vi "Actor Stopped.vi"(8 "error in (no error)":errorcluster, 10 "Actor's Self Q":refnum<class "Message Enqueuer.lvclass">, 11 "Monitor Data in":refnum<class "Monitor Data.lvclass">) -> (0 "error out":errorcluster, 2 "Empty?":bool, 3 "Monitor Data out":refnum<class "Monitor Data.lvclass">)   [LabVIEW 2020, in "Monitor Data.lvclass"]
doc: "Removes the actor from the data store\n\nCopyright: MGI 2016\nAuthor: Derek Trepanier"
uses:
  <vilib>/MGI/Monitored Actor/Monitor Data/Monitor Data.lvclass
  <vilib>/ActorFramework/Message Enqueuer/Message Enqueuer.lvclass
  <vilib>/MGI/Monitored Actor/Monitor Data/Monitor Data.lvclass/Monitor Data.ctl
  <vilib>/MGI/Monitored Actor/Monitor Data/Actor Data.ctl
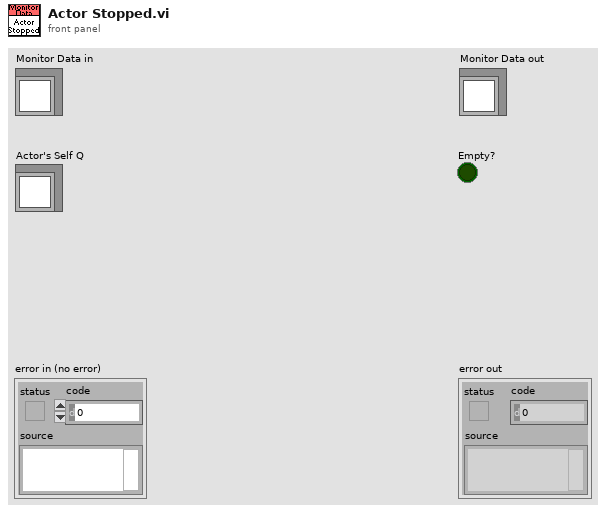
[diagram p1: front panel]
types:
  T1 = typedef "Monitor Data.lvclass/Actor Data.ctl" = cluster{"Actor Type":string, "Actor Core VI":string, "Self":refnum<class "Message Enqueuer.lvclass">, "Caller":refnum<class "Message Enqueuer.lvclass">, "Actor Label":string, "Last Ping":dbl}
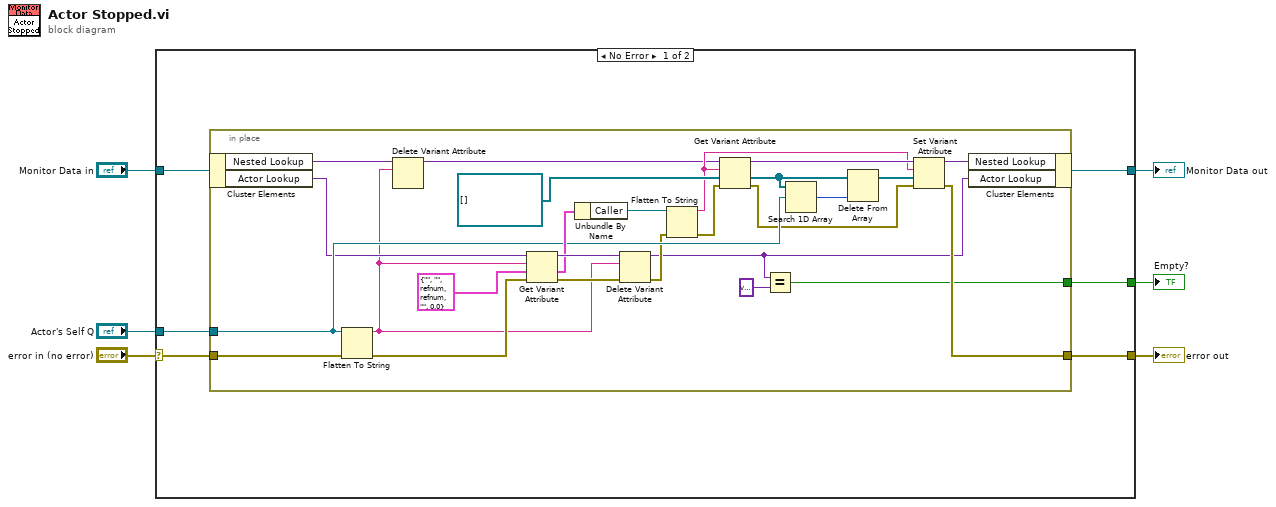
[diagram p0: block diagram]
diagram:
  n1 = case shown="No Error" "error in (no error)" {
    selector: "error in (no error)" -> [w10 w40]
    tunnel: [w9 w40] -> w4
    tunnel: [w8 w39] -> w2
    tunnel: "Monitor Data in" -> [w11 w39]
    tunnel: "Actor's Self Q" -> [w12 _]
    tunnel: [w7 _] -> w1
    frame No Error {
      n2 = in-place {
        in-place-border: w12 -> [w26]
        in-place-border: w10 -> [w19]
        in-place-border: [w18] -> w9
        in-place-border: [w14] -> w7
        n3 = in-place-cluster #1(w11) -> ("Nested Lookup"=w25:variant, "Actor Lookup"=w24:variant)
        n4 = Flatten To String(anything=w26, error in (no error)=w19) -> (data string=w13:string, error out=w37:errorcluster)  [unwired: 2 in, 1 out]
        n5 = Delete Variant Attribute(6:w13, 7:w25) -> (3:w17:variant)  [unwired: 1 in, 2 out]
        n6 = Get Variant Attribute(Variant=w24, name=w13, default value (empty Variant)=T1 {"Actor Type"="", "Actor Core VI"="", "Self"=refnum, "Caller"=refnum, "Actor Label"="", "Last Ping"=0.0} ("Actor Data"), error in=w37) -> (duplicate Variant=w36:variant, value=w34:T1, error out=w35:errorcluster)  [unwired: 1 out]
        n7 = Unbundle By Name(w34) -> ("Caller"=w31:refnum<class "Message Enqueuer.lvclass">)
        n8 = Delete Variant Attribute(4:w35, 6:w13, 7:w36) -> (0:w22:errorcluster, 3:w16:variant)  [unwired: 1 out]
        n9 = Flatten To String(anything=w31, error in (no error)=w22) -> (data string=w28:string, error out=w21:errorcluster)  [unwired: 2 in, 1 out]
        n10 = Get Variant Attribute(Variant=w17, name=w28, default value (empty Variant)=refnum<class "Message Enqueuer.lvclass">[] [], error in=w21) -> (duplicate Variant=w33:variant, value=w30:refnum<class "Message Enqueuer.lvclass">[], error out=w20:errorcluster)  [unwired: 1 out]
        n11 = Equal?(x=w16, y=variant) -> (x = y?=w14:bool)
        n12 = Search 1D Array(1D array=w30, element=w26) -> (index of element=w27:i32)  [unwired: 1 in]
        n13 = Delete From Array(array=w30, index=w27) -> (array with subset deleted=w29:refnum<class "Message Enqueuer.lvclass">[])  [unwired: 1 in, 1 out]
        n14 = Set Variant Attribute(Variant=w33, name=w28, value=w29, error in=w20) -> (Variant out=w23:variant, error out=w18:errorcluster)  [unwired: 1 out]
        n15 = in-place-cluster #1("Nested Lookup"=w23, "Actor Lookup"=w16) -> (w8:refnum<class "Monitor Data.lvclass">)
      }
    }
    frame Error {
    }
  }
  "error out" <- w4
  "Monitor Data out" <- w2
  "Empty?" <- w1
